vi "UnregisterSALEvents.vi"(8 "error in (no error)":errorcluster, 11 "SAL in":refnum<class "SAL.lvclass">) -> (0 "error out":errorcluster, 3 "SAL out":refnum<class "SAL.lvclass">)   [LabVIEW 2016, in "SAL.lvclass"]
uses:
  SAL.lvclass
  SALLV_m1m3/SALLV_m1m3.lvlib
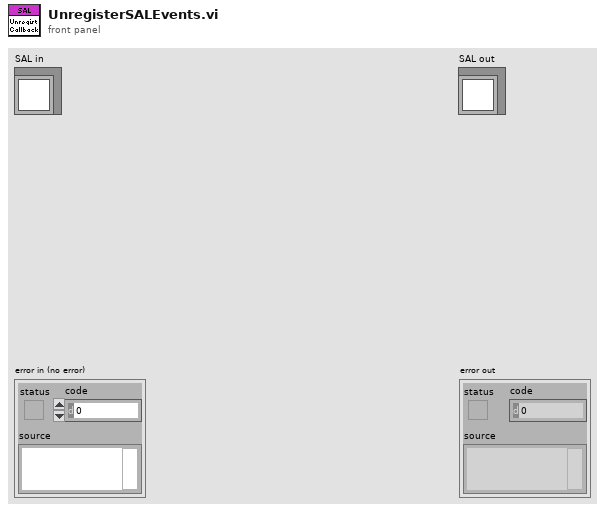
[diagram p1: front panel]
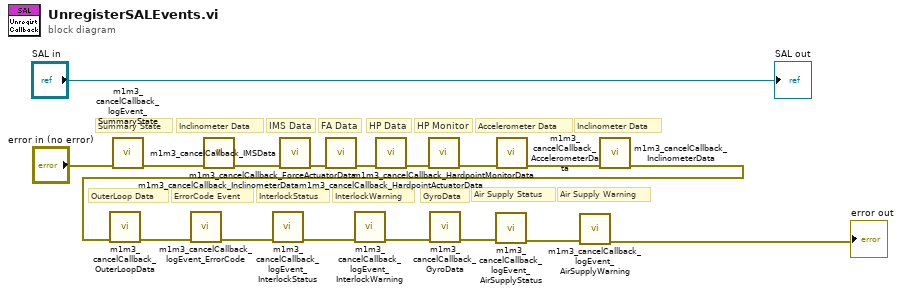
[diagram p0: block diagram]
diagram:
  # "Air Supply Warning"
  # "Air Supply Status"
  # "GyroData"
  # "InterlockWarning"
  # "InterlockStatus"
  # "ErrorCode Event"
  # "OuterLoop Data"
  # "Inclinometer Data"
  # "Accelerometer Data"
  # "HP Monitor"
  # "HP Data"
  # "FA Data"
  # "IMS Data"
  # "Inclinometer Data"
  # "Summary State"
  n1 = call "m1m3_cancelCallback_logEvent_SummaryState.vi"("error in (no error)"="error in (no error)") -> ("error out"=w15:errorcluster)  [unwired: 9 in, 1 out]
  n2 = call "m1m3_cancelCallback_InclinometerData.vi"("error in (no error)"=w15) -> ("error out"=w14:errorcluster)  [unwired: 9 in, 1 out]
  n3 = call "m1m3_cancelCallback_IMSData.vi"("error in (no error)"=w14) -> ("error out"=w13:errorcluster)  [unwired: 9 in, 1 out]
  n4 = call "m1m3_cancelCallback_ForceActuatorData.vi"("error in (no error)"=w13) -> ("error out"=w7:errorcluster)  [unwired: 9 in, 1 out]
  n5 = call "m1m3_cancelCallback_HardpointActuatorData.vi"("error in (no error)"=w7) -> ("error out"=w12:errorcluster)  [unwired: 9 in, 1 out]
  n6 = call "m1m3_cancelCallback_HardpointMonitorData.vi"("error in (no error)"=w12) -> ("error out"=w6:errorcluster)  [unwired: 9 in, 1 out]
  n7 = call "m1m3_cancelCallback_AccelerometerData.vi"("error in (no error)"=w6) -> ("error out"=w11:errorcluster)  [unwired: 9 in, 1 out]
  n8 = call "m1m3_cancelCallback_InclinometerData.vi"("error in (no error)"=w11) -> ("error out"=w4:errorcluster)  [unwired: 9 in, 1 out]
  n9 = call "m1m3_cancelCallback_OuterLoopData.vi"("error in (no error)"=w4) -> ("error out"=w10:errorcluster)  [unwired: 9 in, 1 out]
  n10 = call "m1m3_cancelCallback_logEvent_ErrorCode.vi"("error in (no error)"=w10) -> ("error out"=w9:errorcluster)  [unwired: 9 in, 1 out]
  n11 = call "m1m3_cancelCallback_logEvent_InterlockStatus.vi"("error in (no error)"=w9) -> ("error out"=w8:errorcluster)  [unwired: 9 in, 1 out]
  n12 = call "m1m3_cancelCallback_logEvent_InterlockWarning.vi"("error in (no error)"=w8) -> ("error out"=w5:errorcluster)  [unwired: 9 in, 1 out]
  n13 = call "m1m3_cancelCallback_GyroData.vi"("error in (no error)"=w5) -> ("error out"=w3:errorcluster)  [unwired: 9 in, 1 out]
  n14 = call "m1m3_cancelCallback_logEvent_AirSupplyStatus.vi"("error in (no error)"=w3) -> ("error out"=w2:errorcluster)  [unwired: 9 in, 1 out]
  n15 = call "m1m3_cancelCallback_logEvent_AirSupplyWarning.vi"("error in (no error)"=w2) -> ("error out"=→"error out":errorcluster)  [unwired: 9 in, 1 out]
  "SAL out" <- "SAL in"
